vi "Aperture Server (UCPTWO's conflicted copy 2019-02-19).vi"() -> ()   [LabVIEW 2018]
doc: "Use this VI to connect and control an unknown DC motor stage with the C-843. Select first if the connected stage is analog or PWM driven. The VI runs \"C843_Configuration_Setup.vi\" without moving any axis. It defines axis 1 to be \"DEFAULT_STAGE\" (analog) or \"DEFAULT_STAGE_P\" (PWM), which corresponds to no limit switches, no reference switch, and a position unit of 1 count. It reads the current velocity, the maximum allowed velocity, and the PID values of this stage type and sets the servo state to ON. Then it runs in a loop, reading the current position value, and giving the user the possibility to make relative moves in forward or backward direction, or to set velocity and PID values. Pressing the STOP button will send a STP command to the board, set the servo state to OFF and stop the VI."
panel:
  in  "Type":enum16{"Analog", "PWM"}(ring)
  in  "System no.":i32=1 min=1 step=1
  in  "C-843 Board No.":i32=1 min=0 step=1
  in  "Servo mode":bool=TRUE
  in  "D-Term":dbl=350.0 format="%.6f"
  out "Max Velocity":dbl=100.0 format="%.6f"
  in  "I-Term":dbl=5.0 format="%.6f"
  in  "P-Term":dbl=140.0 format="%.6f"
  in  "Velocity":dbl=10.0 format="%.6f"
  in  "Stop":bool
  in  "Step Size":dbl=100.0 format="%.6f"
  in  "Step Right":bool
  out "Position":dbl format="%.6f"
  in  "Update Parameters":bool
  in  "Step Left":bool
  in  "stop":bool
  in  "error in":errorcluster
  out "error out":errorcluster
  out "Conn. Axis":string[](array[string])
  out "Identification":string
  # "Operation:"
  # "Parameter settings:"
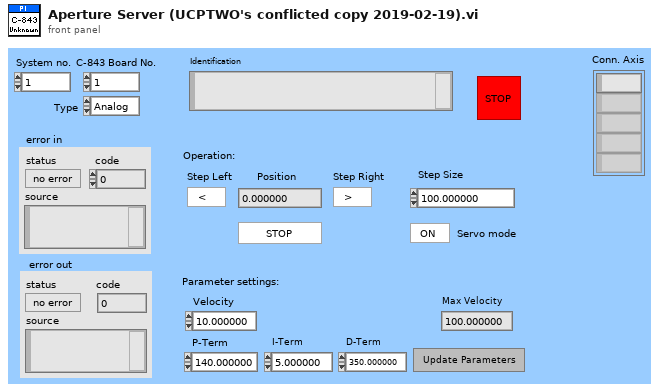
[diagram p1: front panel]
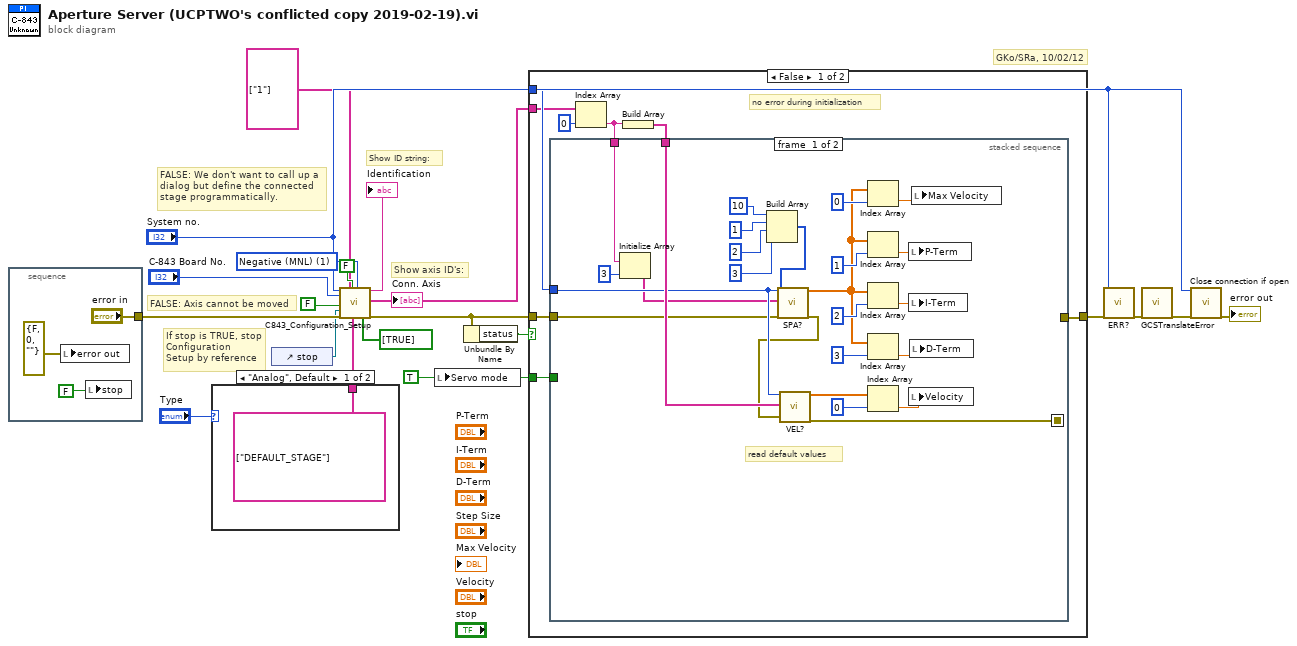
[diagram p0: block diagram]
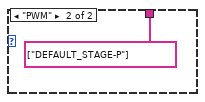
[diagram p2: hidden frame]
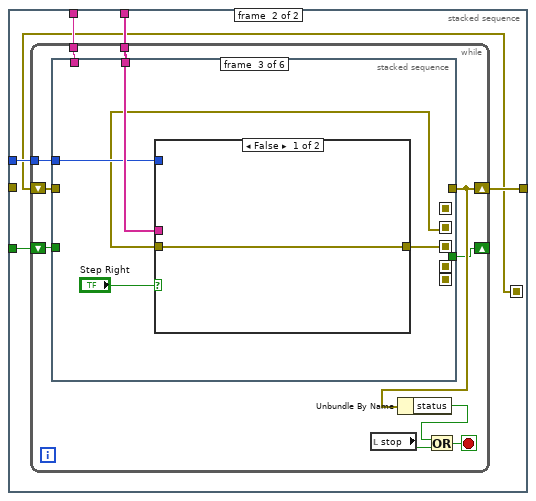
[diagram p3: hidden frame]
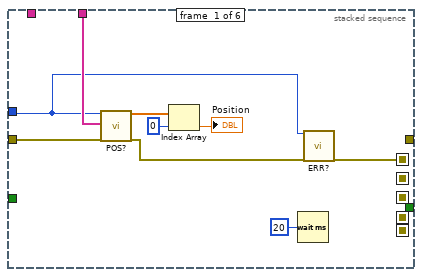
[diagram p4: hidden frame]
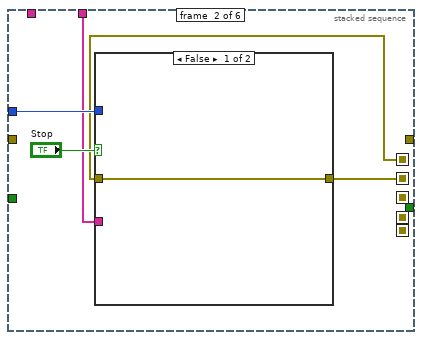
[diagram p5: hidden frame]
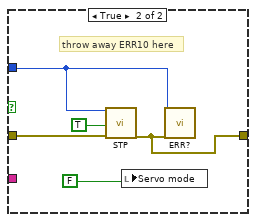
[diagram p6: hidden frame]
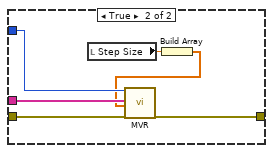
[diagram p7: hidden frame]
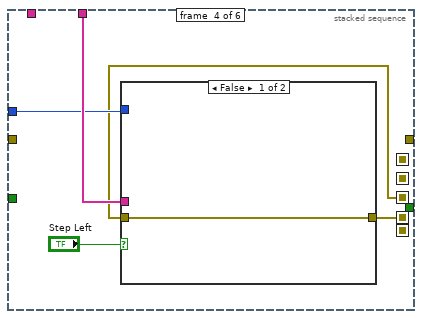
[diagram p8: hidden frame]
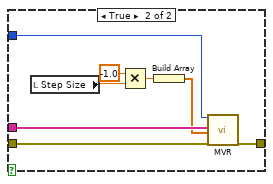
[diagram p9: hidden frame]
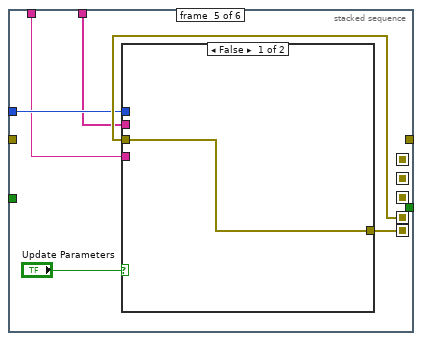
[diagram p10: hidden frame]
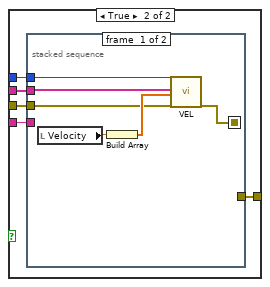
[diagram p11: hidden frame]
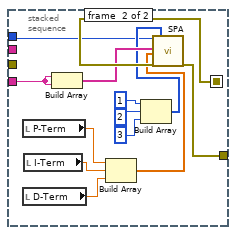
[diagram p12: hidden frame]
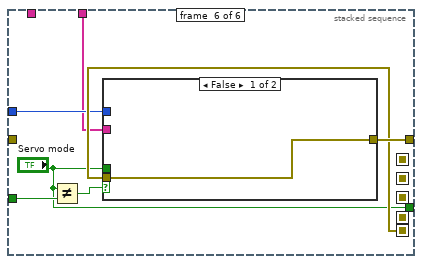
[diagram p13: hidden frame]
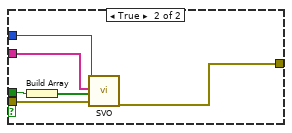
[diagram p14: hidden frame]
diagram:
  w3 = u16 1 items=["Positive (MPL)", "Negative (MNL)"] ("Limit switch selection")
  w9 = TRUE ("Servo mode")
  # "If stop is TRUE, stop \nConfiguration\nSetup by reference"
  # "GKo/SRa, 10/02/12"
  # "Show axis ID's:"
  # "Show ID string:"
  # "FALSE: We don't want to call up a \ndialog but define the connected\nstage programmatically."
  # "FALSE: Axis cannot be moved"
  n1 = stacked-sequence {
    tunnel: ["error in"] -> w18
    frame #0 {
      n2 = local write "error out"(errorcluster {"status"=FALSE, "code"=0, "source"=""} ("error in")) -> ()
      n3 = local write "stop"(FALSE ("stop")) -> ()
    }
  }
  n4 = case shown="\"Analog\", Default" "Type" {
    tunnel: [string[] ["DEFAULT_STAGE"] ("Stage names input") string[] ["DEFAULT_STAGE-P"] ("Stage names input")] -> w11
    frame "Analog", Default {
    }
    frame "PWM" {
    }
  }
  n5 = control-ref of="stop"() -> (w10:refnum<vi>)
  n6 = call "C843_Configuration_Setup.vi"("System no."="System no.", "C-843 Board No."="C-843 Board No.", "All axes?"=FALSE, "Stop refnum"=w10, "error in"=w18, "Use dialog to define\nconnected stages?"=FALSE ("Use dialog to define\nconnected stages?"), "Stage names input"=w11, "Limit switch selection"=w3, "RON Affected axes"=string[] ["1"], "Reference mode"=bool[] [TRUE]) -> ("Identification"=→"Identification":string, "Conn. \nAxes"=w13:string[], "error out"=w16:errorcluster)  [unwired: 5 in, 2 out]
  "Conn. Axis" <- w13
  n7 = local write "Servo mode"(w9) -> ()
  n8 = Unbundle By Name(w16) -> ("status"=w17:bool)
  n9 = case shown="False" w17 {
    tunnel: "System no." -> [w31 _]
    tunnel: w16 -> [w33 w166]
    tunnel: [w32 w166] -> w14
    tunnel: w13 -> [w30 _]
    tunnel: w9 -> [w26 _]
    frame False {
      # "no error during initialization"
      n10 = Index Array(array=w30, index=0) -> (element=w27:string)
      n11 = Build Array(w27) -> (w28:string[])
      n12 = stacked-sequence {
        seq-local: [w48 _] -> [_ w60]
        tunnel: w33 -> [w49 _]
        tunnel: [_ w64] -> w32
        tunnel: w31 -> [w51 w63]
        tunnel: w28 -> [w52 w62]
        tunnel: w27 -> [w40 w61]
        tunnel: w26 -> [_ w59]
        frame #0 {
          # "read default values"
          n13 = Initialize Array(w40, 3 ("dimension size")) -> (w39:string[])
          n14 = Build Array(10 ("element"), 1 ("element"), 2 ("element"), 3 ("element")) -> (w56:i32[])
          n15 = call "SPA?.vi"("System no."=w51, "Axes to query"=w39, "Parameter no."=w56, "error in"=w49) -> ("Parameter value"=w36:dbl[], "error out"=w50:errorcluster)  [unwired: 3 in, 11 out]
          n16 = call "VEL?.vi"("System no."=w51, "Axes to query"=w52, "error in"=w50) -> ("Velocity"=w47:dbl[], "error out"=w48:errorcluster)  [unwired: 2 in, 13 out]
          n17 = Index Array(array=w36, index=0) -> (element=w43:dbl)
          n18 = Index Array(array=w36, index=1) -> (element=w55:dbl)
          n19 = Index Array(array=w36, index=2) -> (element=w41:dbl)
          n20 = Index Array(array=w36, index=3) -> (element=w34:dbl)
          n21 = Index Array(array=w47, index=0) -> (element=w46:dbl)
          n22 = local write "P-Term"(w55) -> ()
          n23 = local write "I-Term"(w41) -> ()
          n24 = local write "Velocity"(w46) -> ()
          n25 = local write "D-Term"(w34) -> ()
          n26 = local write "Max Velocity"(w43) -> ()
        }
        frame #1 {
          n27 = while {
            shift-right: [w71] -> w64
            shift-left: w60 -> [w74]
            tunnel: w63 -> [w72]
            tunnel: w62 -> [w73]
            tunnel: w61 -> [w67]
            shift-right: [w65] -> _
            shift-left: w59 -> [w66]
            stop <- w70 stop-if-true
            n28 = stacked-sequence {
              seq-local: [w77 _ _ _ _ _] -> [_ w86 _ _ _ _]
              seq-local: [_ w85 _ _ _ _] -> [_ _ w95 _ _ _]
              seq-local: [_ _ w96 _ _ _] -> [_ _ _ w108 _ _]
              seq-local: [_ _ _ w107 _ _] -> [_ _ _ _ w125 _]
              seq-local: [_ _ _ _ w121 _] -> [_ _ _ _ _ w155]
              tunnel: w74 -> [w83 _ _ _ _ _]
              tunnel: w73 -> [w82 w84 w98 w111 w123 w153]
              tunnel: w72 -> [w75 w87 w97 w110 w124 w154]
              tunnel: [_ _ _ _ _ w156] -> w71
              tunnel: w67 -> [_ _ _ _ w122 _]
              tunnel: w66 -> [_ _ _ _ _ w158]
              tunnel: [_ _ _ _ _ "Servo mode"] -> w65
              frame #0 {
                n29 = call "POS?.vi"("System no."=w75, "Axes to query"=w82, "error in"=w83) -> ("Position"=w81:dbl[], "error out"=w76:errorcluster)  [unwired: 2 in, 13 out]
                n30 = Index Array(array=w81, index=0) -> (element=→"Position":dbl)
                n31 = Wait (ms)(milliseconds to wait=u32 20) -> ()  [unwired: 1 out]
                n32 = call "ERR?.vi"("System no."=w75, "error in"=w76) -> ("error out"=w77:errorcluster)  [unwired: 17 out]
              }
              frame #1 {
                n33 = case shown="False" "Stop" {
                  tunnel: w87 -> [_ w92]
                  tunnel: w86 -> [w89 w94]
                  tunnel: [w89 w91] -> w85
                  tunnel: w84 -> [_ _]
                  frame False {
                  }
                  frame True {
                    # "throw away ERR10 here"
                    n34 = call "STP.vi"("System no."=w92, "All axes?"=TRUE, "error in"=w94) -> ("error out"=w91:errorcluster)  [unwired: 2 in, 14 out]
                    n35 = local write "Servo mode"(FALSE ("Servo mode")) -> ()
                    n36 = call "ERR?.vi"("System no."=w92, "error in"=w91) -> ()  [unwired: 18 out]
                  }
                }
              }
              frame #2 {
                n37 = case shown="False" "Step Right" {
                  tunnel: w98 -> [_ w105]
                  tunnel: w97 -> [_ w106]
                  tunnel: w95 -> [w100 w104]
                  tunnel: [w100 w103] -> w96
                  frame False {
                  }
                  frame True {
                    n38 = local read "Step Size"() -> (w102:dbl)
                    n39 = Build Array(w102) -> (w101:dbl[])
                    n40 = call "MVR.vi"("System no."=w106, "Axes to move"=w105, "Position values"=w101, "error in"=w104) -> ("error out"=w103:errorcluster)  [unwired: 1 in, 14 out]
                  }
                }
              }
              frame #3 {
                n41 = case shown="False" "Step Left" {
                  tunnel: w111 -> [_ w119]
                  tunnel: w110 -> [_ w120]
                  tunnel: w108 -> [w112 w118]
                  tunnel: [w112 w117] -> w107
                  frame False {
                  }
                  frame True {
                    n42 = local read "Step Size"() -> (w113:dbl)
                    n43 = Multiply(x=-1.0, y=w113) -> (x*y=w115:dbl)
                    n44 = Build Array(w115) -> (w116:dbl[])
                    n45 = call "MVR.vi"("System no."=w120, "Axes to move"=w119, "Position values"=w116, "error in"=w118) -> ("error out"=w117:errorcluster)  [unwired: 1 in, 14 out]
                  }
                }
              }
              frame #4 {
                n46 = case shown="False" "Update Parameters" {
                  tunnel: w125 -> [w127 w130]
                  tunnel: w124 -> [_ w132]
                  tunnel: w123 -> [_ w131]
                  tunnel: w122 -> [_ w129]
                  tunnel: [w127 w128] -> w121
                  frame False {
                  }
                  frame True {
                    n47 = stacked-sequence {
                      seq-local: [w133 _] -> [_ w151]
                      tunnel: w132 -> [w138 w142]
                      tunnel: w131 -> [w137 _]
                      tunnel: w130 -> [w135 _]
                      tunnel: w129 -> [_ w147]
                      tunnel: [_ w139] -> w128
                      frame #0 {
                        n48 = local read "Velocity"() -> (w134:dbl)
                        n49 = Build Array(w134) -> (w136:dbl[])
                        n50 = call "VEL.vi"("System no."=w138, "Axes to set"=w137, "Velocity values"=w136, "error in"=w135) -> ("error out"=w133:errorcluster)  [unwired: 2 in, 13 out]
                      }
                      frame #1 {
                        n51 = local read "P-Term"() -> (w149:dbl)
                        n52 = local read "D-Term"() -> (w140:dbl)
                        n53 = local read "I-Term"() -> (w148:dbl)
                        n54 = Build Array(w147, w147) -> (w146:string[])
                        n55 = Build Array(w149, w148, w140) -> (w150:dbl[])
                        n56 = Build Array(1 ("element"), 2 ("element"), 3 ("element")) -> (w145:i32[])
                        n57 = call "SPA.vi"("System no."=w142, "Axis to set"=w146, "Parameter value"=w150, "error in"=w151, "Parameter number"=w145) -> ("error out"=w139:errorcluster)  [unwired: 5 in, 9 out]
                      }
                    }
                  }
                }
              }
              frame #5 {
                n58 = Not Equal?(x="Servo mode", y=w158) -> (x != y?=w157:bool)
                n59 = case shown="False" w157 {
                  tunnel: "Servo mode" -> [_ w165]
                  tunnel: [w159 w163] -> w156
                  tunnel: w155 -> [w159 w162]
                  tunnel: w154 -> [_ w161]
                  tunnel: w153 -> [_ w160]
                  frame False {
                  }
                  frame True {
                    n60 = Build Array(w165) -> (w164:bool[])
                    n61 = call "SVO.vi"("System no."=w161, "Axes to command"=w160, "Servo mode"=w164, "error in"=w162) -> ("error out"=w163:errorcluster)  [unwired: 1 in, 14 out]
                  }
                }
              }
            }
            n62 = local read "stop"() -> (w69:bool)
            n63 = Unbundle By Name(w71) -> ("status"=w68:bool)
            n64 = Or(x=w68, y=w69) -> (x .or. y?=w70:bool)
          }
        }
      }
    }
    frame True {
      # "error during initialization!"
    }
  }
  n65 = call "ERR?.vi"("System no."="System no.", "error in"=w14) -> ("error out"=w15:errorcluster)  [unwired: 17 out]
  n66 = call "GCSTranslateError.vi"("error in"=w15) -> ("error out"=w8:errorcluster)  [unwired: 18 out]
  n67 = call "Close connection if open.vi"("System no."="System no.", "error in"=w8) -> ("error out"=→"error out":errorcluster)  [unwired: 1 in, 16 out]
